vi "locate seq channel to modify.vi"(7 "owner ID":string, 8 "error in":errorcluster, 10 "tag descriptor":refnum<class "tag descriptor.lvclass">, 11 "engine configuration in":refnum<class "base TBM sequencer configuration.lvclass">) -> (0 "error out":errorcluster, 2 "index":i32, 3 "engine configuration out":refnum<class "base TBM sequencer configuration.lvclass">)   [LabVIEW 2014, in "base TBM sequencer configuration.lvclass"]
uses:
  base TBM sequencer configuration.lvclass
  <vilib>/NI/Tag Bus/tag/tag descriptor.lvclass
  <vilib>/NI/Configuration Framework/NISE_CEF_TreeControl.lvlib
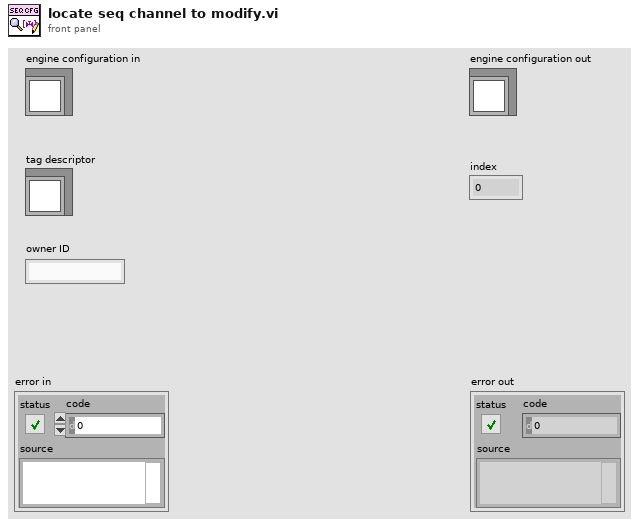
[diagram p1: front panel]
types:
  T1 = typedef "base TBM sequencer configuration.lvclass/Tag Info.ctl" = cluster{"Channel":refnum<class "TBM channel.lvclass">, "Writers":string[], "Readers":string[], "Owning ID":string}
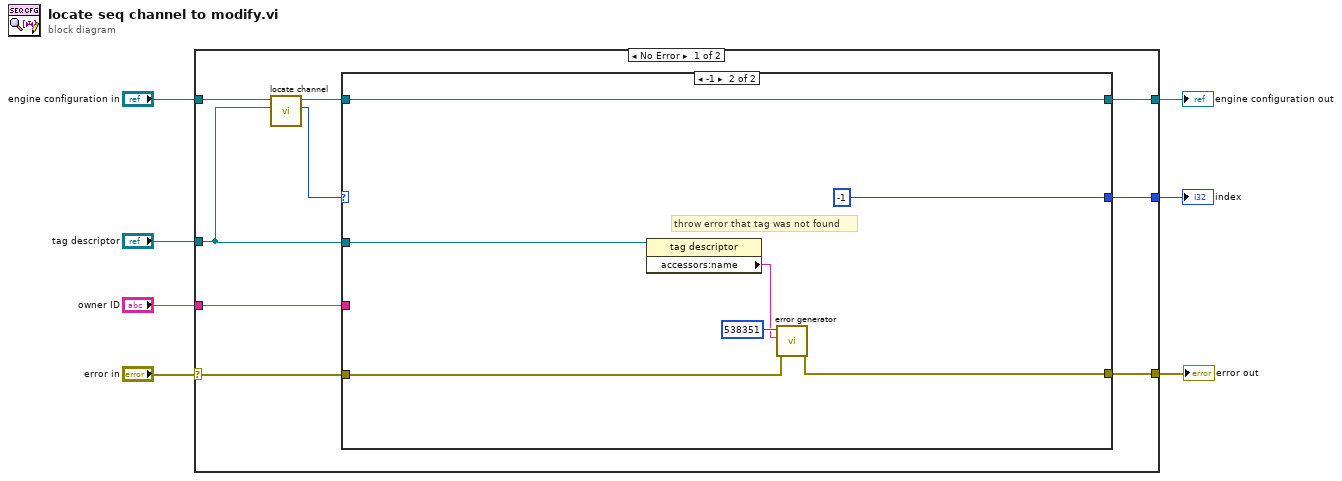
[diagram p0: block diagram]
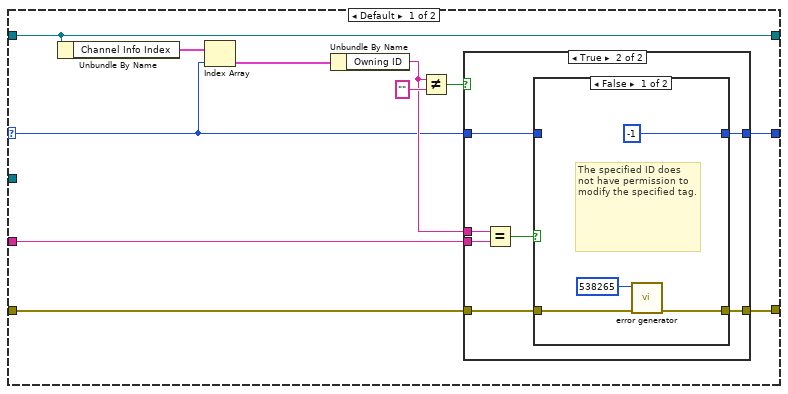
[diagram p2: hidden frame]
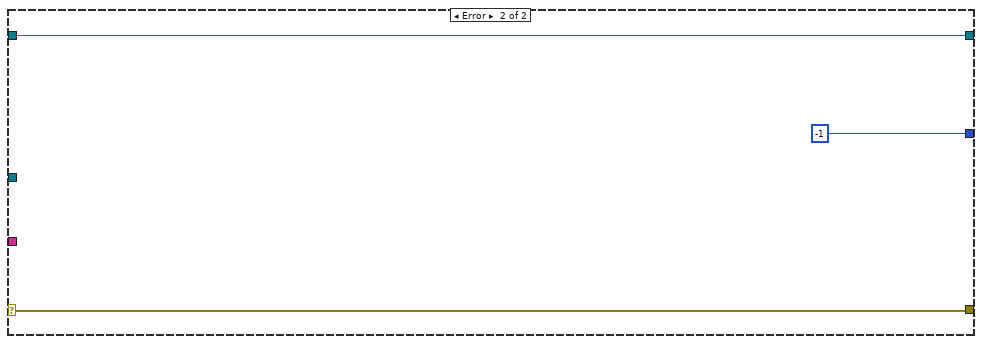
[diagram p5: hidden frame]
diagram:
  n1 = case shown="No Error" "error in" {
    selector: "error in" -> [w12 w50]
    tunnel: "engine configuration in" -> [w16 w52]
    tunnel: [w13 w52] -> w6
    tunnel: "tag descriptor" -> [w11 _]
    tunnel: [w10 w50] -> w3
    tunnel: "owner ID" -> [w9 _]
    tunnel: [w8 -1 ("index")] -> w1
    frame No Error {
      n2 = call "locate channel.vi"("tag descriptor"=w11, "sequencer config in"=w16) -> ("index"=w15:i32, "sequencer config out"=w14:refnum<class "base TBM sequencer configuration.lvclass">)  [unwired: 8 in]
      n3 = case shown="-1" w15 {
        selector: w15 -> [w18 _]
        tunnel: w14 -> [w20 w49]
        tunnel: [w20 w49] -> w13
        tunnel: w12 -> [w22 w47]
        tunnel: w11 -> [_ w46]
        tunnel: [w21 w44] -> w10
        tunnel: w9 -> [w24 _]
        tunnel: [w23 -1 ("index")] -> w8
        frame Default {
          n4 = Unbundle By Name(w20) -> ("Channel Info Index"=w19:T1[])
          n5 = Index Array(array=w19, index=w18) -> (element=w17:T1)
          n6 = Unbundle By Name(w17) -> ("Owning ID"=w25:string)
          n7 = Not Equal?(x=w25, y="") -> (x != y?=w26:bool)
          n8 = case shown="True" w26 {
            tunnel: w25 -> [_ w35]
            tunnel: w24 -> [_ w36]
            tunnel: w18 -> [w29 w34]
            tunnel: [w29 w33] -> w23
            tunnel: w22 -> [w28 w32]
            tunnel: [w28 w30] -> w21
            frame False {
            }
            frame True {
              n9 = Equal?(x=w35, y=w36) -> (x = y?=w31:bool)
              n10 = case shown="False" w31 {
                tunnel: w34 -> [_ w42]
                tunnel: [-1 ("index") w42] -> w33
                tunnel: w32 -> [w38 w41]
                tunnel: [w37 w41] -> w30
                frame False {
                  # "The specified ID does not have permission to modify the specified tag."
                  n11 = call <vilib>:"error generator.vi"("error in"=w38, "error code (0)"=538265) -> ("error out"=w37:errorcluster)  [unwired: 7 in]
                }
                frame True {
                }
              }
            }
          }
        }
        frame -1 {
          # "throw error that tag was not found"
          n12 = property class="tag descriptor"(reference=w46) -> ("accessors:name"=w45:string)  [unwired: 1 in, 2 out]
          n13 = call <vilib>:"error generator.vi"("error in"=w47, "append error message"=w45, "error code (0)"=538351) -> ("error out"=w44:errorcluster)  [unwired: 6 in]
        }
      }
    }
    frame Error {
    }
  }
  "engine configuration out" <- w6
  "index" <- w1
  "error out" <- w3
